vi "Write Multi Variant as Value.vi"(8 "error in (no error)":errorcluster, 9 "Array":variant[](array[variant]), 10 "Tag":string[](array[string]), 11 "Var Bus in":refnum<class "Omni_Bus.lvclass">) -> (0 "error out":errorcluster, 3 "Var Bus out":refnum<class "Omni_Bus.lvclass">)   [LabVIEW 2021, in "Omni_Bus.lvclass"]
uses:
  Omni_Bus.lvclass
  <vilib>/TSA/Abstract Data Classes/Abs_Types/Value/Abs_Value.lvclass
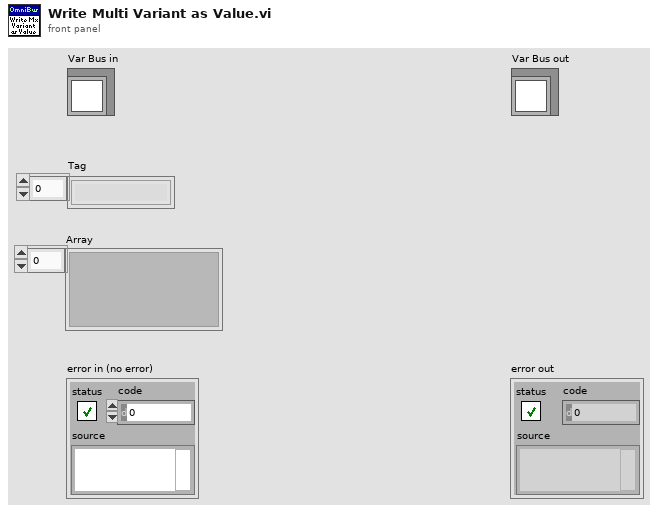
[diagram p1: front panel]
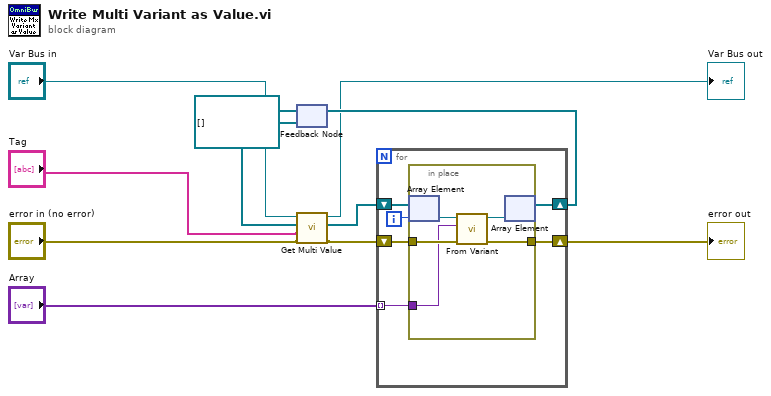
[diagram p0: block diagram]
diagram:
  n1 = feedback #1(refnum<class "Abs_Value.lvclass">[] []) -> (w5:refnum<class "Abs_Value.lvclass">[])
  n2 = call-dynamic "Get Multi Value.vi"("error in (no error)"="error in (no error)", "Tag"="Tag", "Value Type"=w5, "Var Bus in"="Var Bus in") -> ("error out"=w9:errorcluster, "Value Out"=w8:refnum<class "Abs_Value.lvclass">[], "Var Bus out"=→"Var Bus out":refnum<class "Omni_Bus.lvclass">)  [unwired: 4 in, 1 out]
  n3 = for {
    tunnel: "Array" -> [w15] mode=indexing
    shift-right: [w17] -> w11
    shift-left: w9 -> [w16]
    shift-right: [w13] -> w10
    shift-left: w8 -> [w14]
    i -> [w12]
    n4 = in-place {
      in-place-border: [w22] -> w17
      in-place-border: w16 -> [w21]
      in-place-border: w15 -> [w20]
      n5 = in-place-array #2(w14, w12) -> (w19:refnum<class "Abs_Value.lvclass">)
      n6 = call-dynamic "From Variant.vi"("error in (no error)"=w21, "Variant"=w20, "Abs_Value in"=w19) -> ("error out"=w22:errorcluster, "Abs_Value out"=w18:refnum<class "Abs_Value.lvclass">)  [unwired: 7 in]
      n7 = in-place-array #2(w18) -> (w13:refnum<class "Abs_Value.lvclass">[])  [unwired: 1 out]
    }
  }
  "error out" <- w11
  n8 = feedback-in #1(w10) -> ()
